vi "Test Information Dialog.vi"(11 "error in":errorcluster, 12 "Part Numbers":string[](array[string])) -> (1 "Temp  Out":dbl format="%.1g °F", 3 "Specific Gravity Out":dbl format="%.3g", 4 "Parameter Table Out":string[][](table) caption="Parameter Table + Comment Out", 6 "Report Template":path, 10 "Config Path":path, 14 "Part Number 2":u16(ring) items=["2718832", "2718832OLD", "2718834", "3876077-10", "3882506-3", "3882506-5", "3882506-6", "3882842-4", "3882842-5", "3883255-3", "TM Test Bench ini example"], 15 "error out":errorcluster)   [LabVIEW 2018]
doc: "<b>This a dialog box for collecting information from the Operator prior to a new test of a Device/Card/Unit.</b>\n\nThe fields are all alpha-numeric text and are presented in a table. The parameter names are supplied by the calling VI as a 1D array. The results, including the Comment field are returned as a 2D text table, with the parameter names in the first (leftmost) column, and the Operator responses in the second.\n\nNOTE: There is a flat, transparent decoration box covering the left parameter names column to prevent having the Operator change those names at run time.\n\n\nCopyright 2010 Michael Ashe, Imaginatics\n(michael.ashe@imaginatics.net)"
panel:
  in  "Test Comment":string
  in  "Serial Number":string
  in  "Temp":dbl=60.0 format="%.1g °F"
  in  "SG Cal Fluid":dbl format="%#.6g"
  in  "Job Number":string
  in  "Operator Name":string
  in  "Part Number":u16(ring) items=["2718832", "2718832OLD", "2718834", "3876077-10", "3882506-3", "3882506-5", "3882506-6", "3882842-4", "3882842-5", "3883255-3", "TM Test Bench ini example"]
  in  "Cancel":bool
  in  "OK":bool
  # "Test Information"
  # "@"
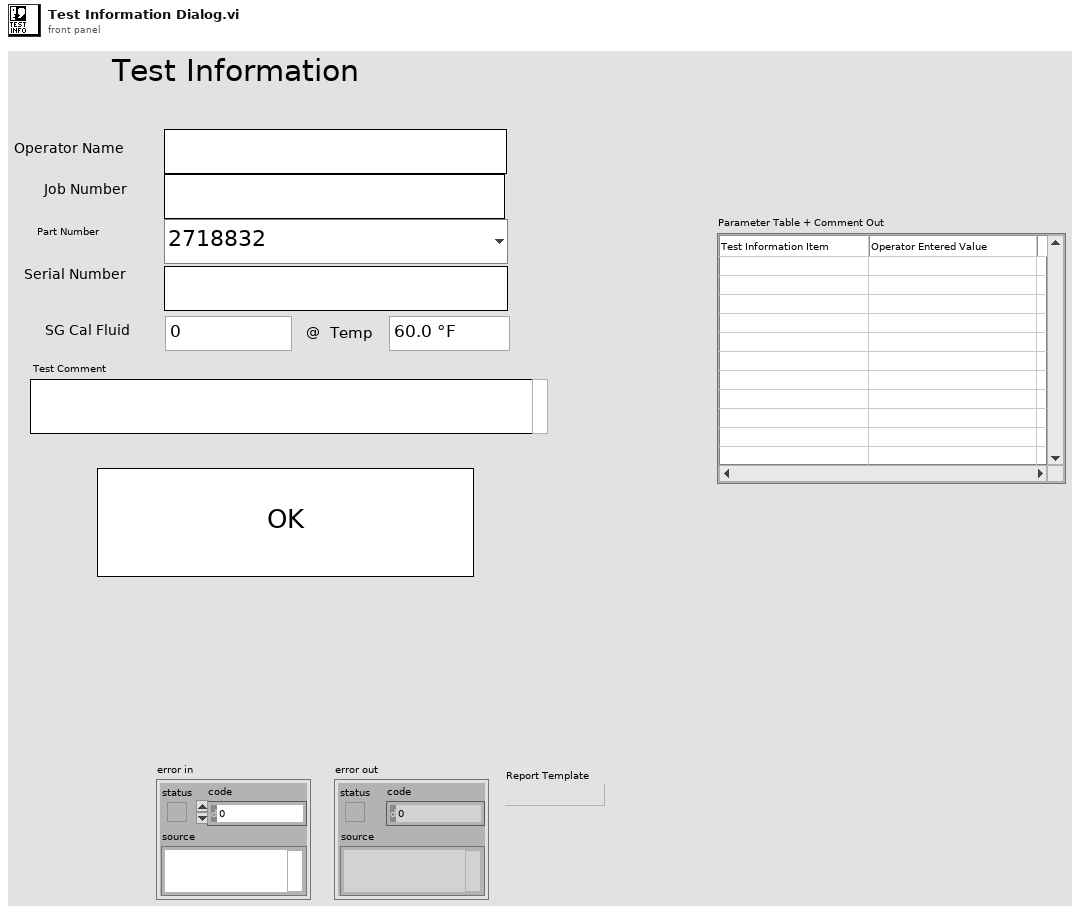
[diagram p1: front panel]
types:
  T1 = enum8{"Enabled", "Disabled", "Disabled and Grayed Out"}
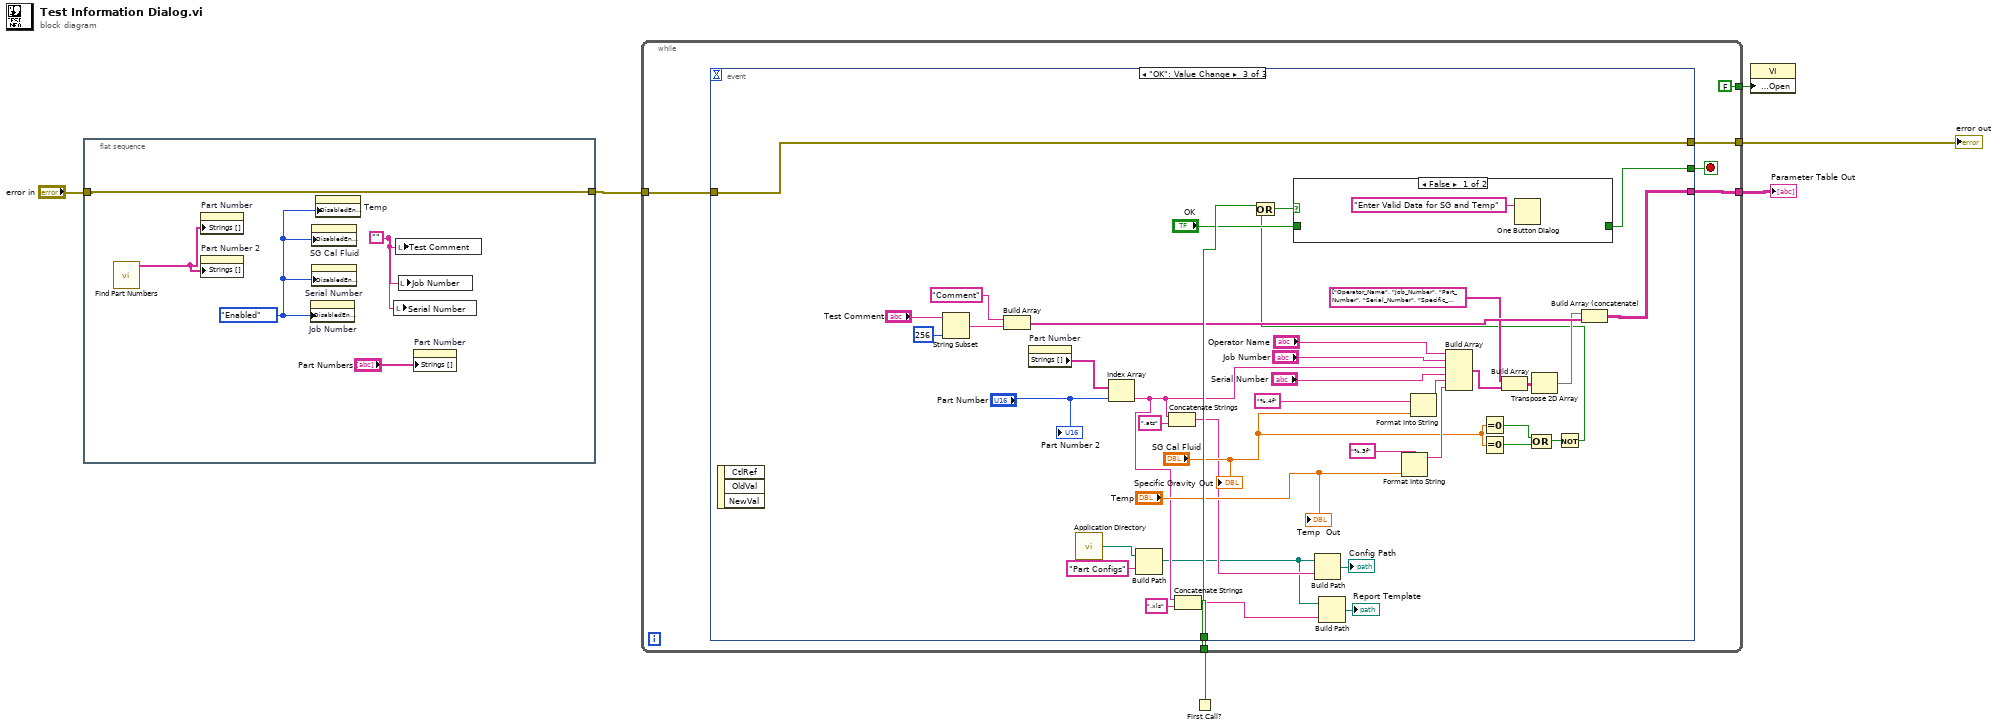
[diagram p0: block diagram]
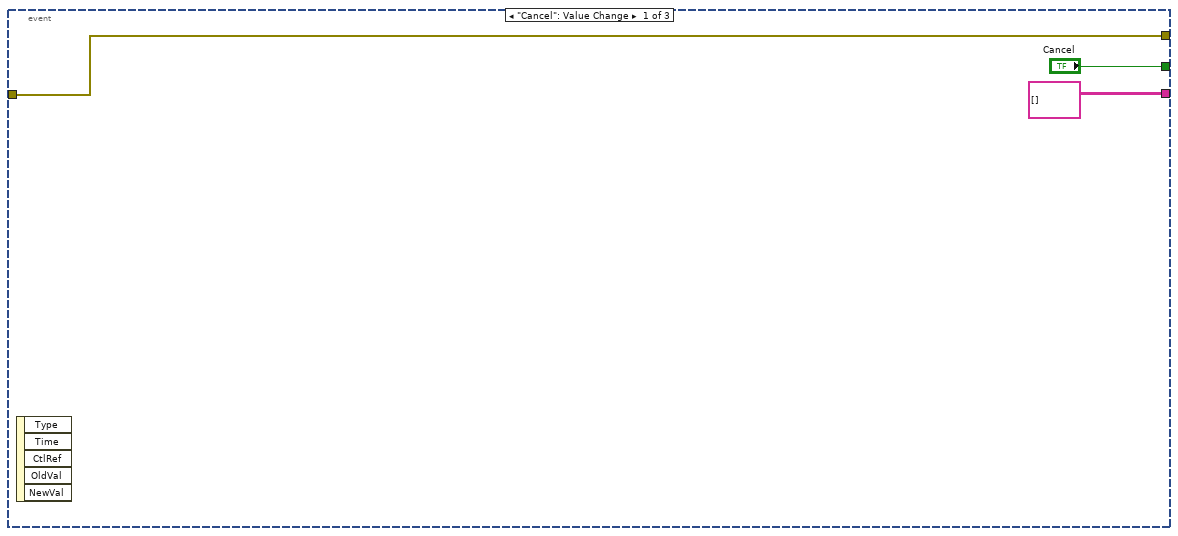
[diagram p2: hidden frame]
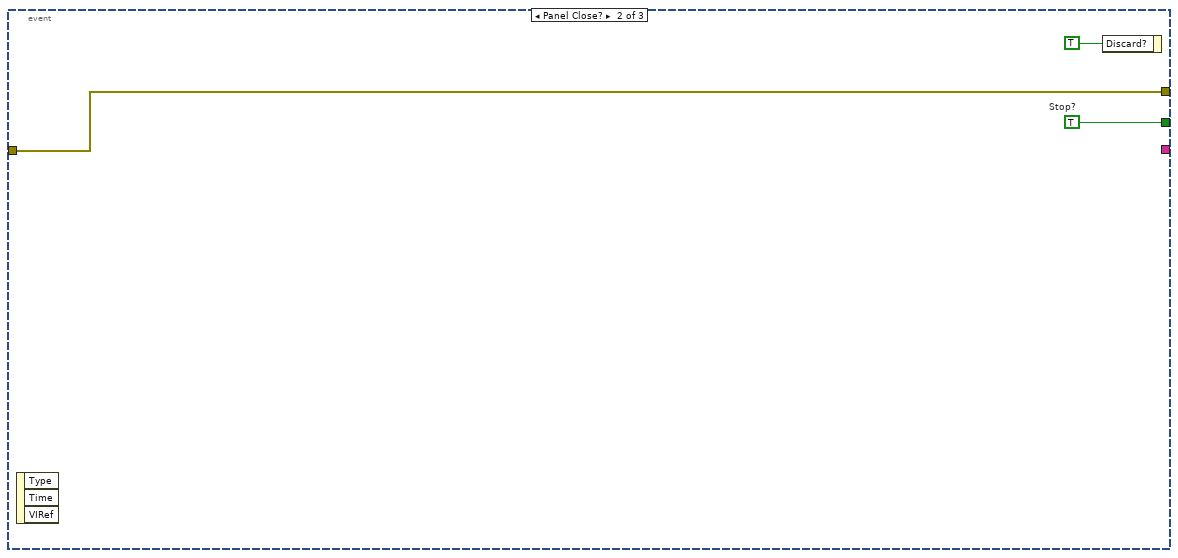
[diagram p3: hidden frame]
diagram:
  n1 = flat-sequence {
    tunnel: [w7] -> w4
    tunnel: "error in" -> [w7]
    frame #0 {
      w8 = T1."Enabled" ("Disabled")
      w10 = ""
      n2 = call "Find Part Numbers.vi"() -> ("Part Numbers"=w9:string[])  [unwired: 11 in]
      n3 = property on="Part Number" class="Ring (strict)"("Strings []"=w9) -> ()  [unwired: 2 in, 2 out]
      n4 = property on="Part Number 2" class="Ring (strict)"("Strings []"=w9) -> ()  [unwired: 2 in, 2 out]
      n5 = property on="Job Number" class="Str"("DisabledEnum"=w8) -> ()  [unwired: 2 in, 2 out]
      n6 = property on="SG Cal Fluid" class="DigNum (strict)"("DisabledEnum"=w8) -> ()  [unwired: 2 in, 2 out]
      n7 = property on="Serial Number" class="Str"("DisabledEnum"=w8) -> ()  [unwired: 2 in, 2 out]
      n8 = property on="Temp" class="DigNum (strict)"("DisabledEnum"=w8) -> ()  [unwired: 2 in, 2 out]
      n9 = local write "Serial Number"(w10) -> ()
      n10 = local write "Test Comment"(w10) -> ()
      n11 = local write "Job Number"(w10) -> ()
      n12 = property on="Part Number" class="Ring (strict)"("Strings []"="Part Numbers") -> ()  [unwired: 2 in, 2 out]
    }
  }
  n13 = First Call?() -> (First Call?: T/F=w2:bool)
  n14 = while {
    tunnel: [w15] -> w6
    tunnel: [w17] -> w5
    tunnel: w2 -> [w14]
    tunnel: w4 -> [w13]
    tunnel: [FALSE ("Front Panel Window:Open")] -> w1
    stop <- w16 stop-if-true
    n15 = event shown="[2] \"OK\": Value Change" {
      selector: _ -> [_ _ _]
      dyn-events: _ -> [_ _ _]
      timeout: _ -> [_ _ _]
      tunnel: [string[][] [] ("Parameter Table 2") _ w63] -> w17
      tunnel: ["Cancel" w23 w61] -> w16
      tunnel: w13 -> [w18 w21 w62]
      tunnel: [w18 w21 w62] -> w15
      tunnel: w14 -> [_ _ w60]
      event "Cancel": Value Change {
        n16 = event-data() -> ()  [unwired: 1 in, 5 out]
      }
      event Panel Close? {
        w23 = TRUE  # Stop?
        n17 = event-data() -> ()  [unwired: 1 in, 3 out]
        n18 = event-data("Discard?"=TRUE) -> ()  [unwired: 1 in, 1 out]
      }
      event "OK": Value Change {
        n19 = event-data() -> ()  [unwired: 1 in, 3 out]
        n20 = String Subset(string="Test Comment", length (rest)=256 ("length (rest)")) -> (substring=w58:string)  [unwired: 1 in]
        n21 = Build Array("Comment", w58) -> (w57:string[])
        n22 = property on="Part Number" class="Ring (strict)"() -> ("Strings []"=w54:string[])  [unwired: 2 in, 2 out]
        n23 = call <vilib>:"Application Directory.vi"() -> ("Application Directory"=w32:path)
        n24 = Index Array(array=w54, index="Part Number") -> (element=w27:string)
        n25 = Build Path(base path=w32, name or relative path="Part Configs") -> (appended path=w26:path)
        n26 = Concatenate Strings(w27, ".ats" ("string")) -> (w33:string)
        n27 = Concatenate Strings(w27, ".xls" ("string")) -> (w25:string)
        n28 = Build Path(base path=w26, name or relative path=w33) -> (appended path=→"Config Path":path)
        n29 = Build Path(base path=w26, name or relative path=w25) -> (appended path=→"Report Template":path)
        n30 = Format Into String(format string="%.3f", "Temp") -> (resulting string=w43:string)  [unwired: 2 in, 1 out]
        n31 = Format Into String(format string="%.4f", "SG Cal Fluid") -> (resulting string=w46:string)  [unwired: 2 in, 1 out]
        n32 = Build Array("Operator Name", "Job Number", w27, "Serial Number", w46, w43) -> (w49:string[])
        n33 = Equal To 0?(x="SG Cal Fluid") -> (x = 0?=w41:bool)
        n34 = Equal To 0?(x="SG Cal Fluid") -> (x = 0?=w40:bool)
        n35 = Build Array(string[] ["Operator_Name", "Job_Number", "Part_Number", "Serial_Number", "Specific_Gravity", "Initial_Temp"] ("ParameterNamesIn 2"), w49) -> (w48:string[][])
        n36 = Transpose 2D Array(2D array=w48) -> (transposed array=w37:string[][])
        n37 = Compound Arithmetic op=OR(w41, w40) -> (w39:bool)
        n38 = Not(x=w39) -> (.not. x?=w36:bool)
        n39 = Or(x=w60, y=w36) -> (x .or. y?=w35:bool)
        n40 = case shown="False" w35 {
          tunnel: "OK" -> [_ w65]
          tunnel: [_ w65] -> w61
          frame False {
            n41 = One Button Dialog(message="Enter Valid Data for SG and Temp") -> ()  [unwired: 1 in, 1 out]
          }
          frame True {
          }
        }
        n42 = Build Array (concatenate)(w37, w57) -> (w63:string[][])
        "Temp  Out" <- "Temp"
        "Specific Gravity Out" <- "SG Cal Fluid"
        "Part Number 2" <- "Part Number"
      }
    }
  }
  "error out" <- w6
  "Parameter Table Out" <- w5
  n43 = property class="VI"("Front Panel.Open"=w1) -> ()  [unwired: 2 in, 2 out]
